vi "BLM Control Com.vi"(1 "command text in":string[](array[string]), 2 "option":T2) -> (0 "Command text out":string[][](array[string]))   [LabVIEW 2024]
uses:
  Ctl/option.ctl
  BLM Control.ctl
panel:
  in  "BLM Control":T1={"extra wait"=0, "Stepper Value"=1e-09, "Value 1"=1.0, "Value 2"=1.0, "String 1"="", "String 2"=""} {"Value 2" format="%#_6e"; "Value 1" format="%<%H:%M:%S>t"; "extra wait" min=0; "Stepper Value" step=0.045 format="%#.7e"}
  in  "cancel":bool
  in  "enter":bool
  # "BLM (Brushless Motor) Control"
  # "(BLM_ManualControl.vi needs to be open before using this program)"
  # "Distance:"
  # "deg of BLM:"
  # "seconds"
  # "AND wait extra"
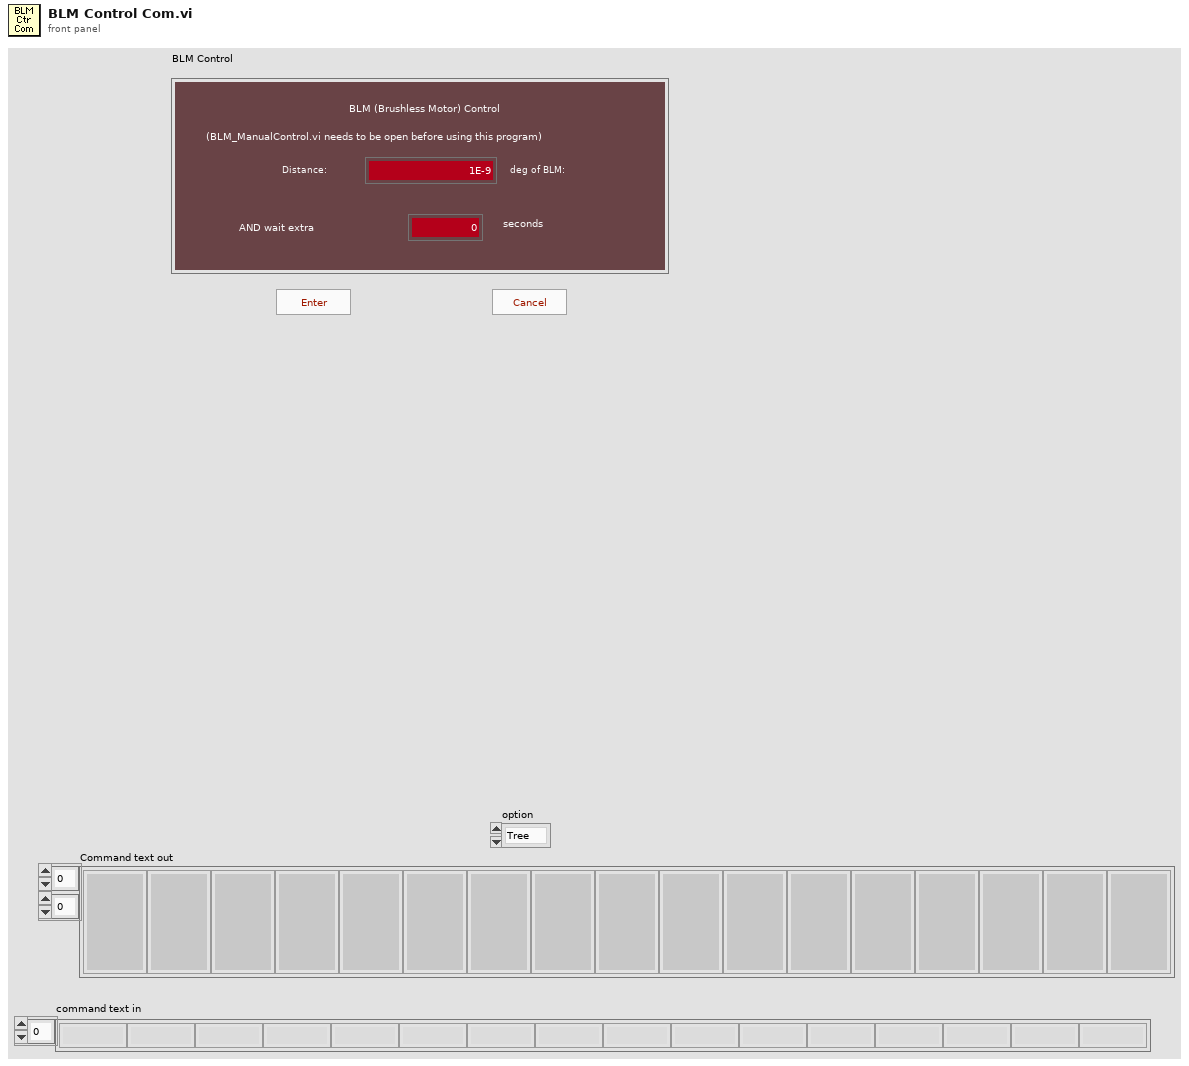
[diagram p1: front panel]
types:
  T1 = typedef "BLM Control.ctl" = cluster{"extra wait":i32, "Stepper Value":dbl, "Value 1":dbl, "Value 2":dbl, "String 1":string, "String 2":string}
  T2 = typedef "option.ctl" = enum16{"Tree", "List"}
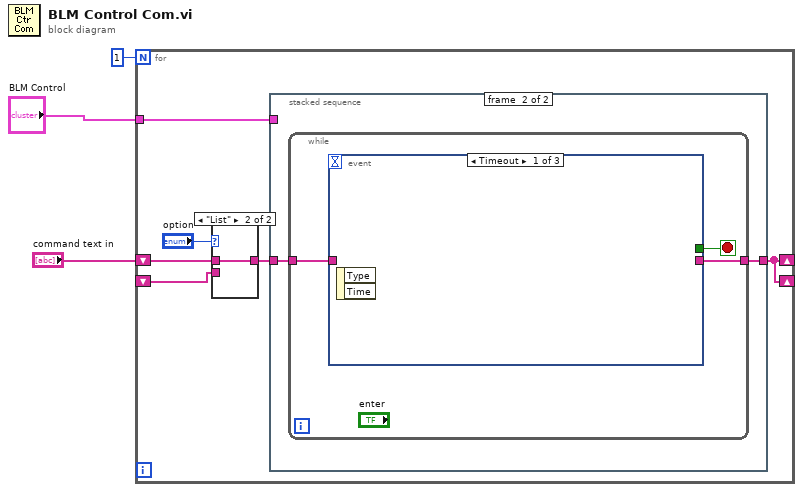
[diagram p0: block diagram]
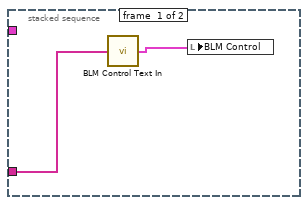
[diagram p3: hidden frame]
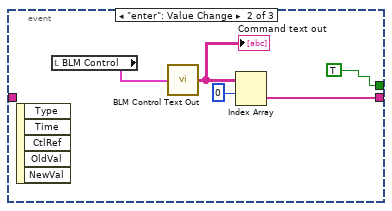
[diagram p4: hidden frame]
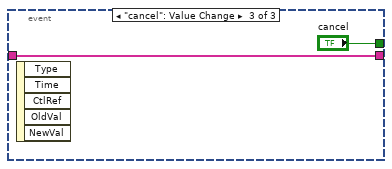
[diagram p5: hidden frame]
diagram:
  n1 = for {
    N: 1 -> [_]
    shift-right: [w4] -> _
    shift-left: _ -> [w8]
    shift-right: [w4] -> _
    shift-left: "command text in" -> [w7]
    tunnel: "BLM Control" -> [w5]
    n2 = case shown="\"List\"" "option" {
      tunnel: [w10 w11] -> w9
      tunnel: w8 -> [w10 _]
      tunnel: w7 -> [_ w11]
      frame "Tree", Default {
      }
      frame "List" {
      }
    }
    n3 = stacked-sequence {
      tunnel: [_ w15] -> w4
      tunnel: w9 -> [w12 w14]
      tunnel: w5 -> [_ _]
      frame #0 {
        n4 = call "BLM Control Text In.vi"("command text in"=w12) -> ("BLM Control"=w13:T1)
        n5 = local write "BLM Control"(w13) -> ()
      }
      frame #1 {
        n6 = while {
          tunnel: [w17] -> w15
          tunnel: w14 -> [w16]
          stop <- w18 stop-if-true
          n7 = event shown="[0] Timeout" {
            selector: _ -> [_ _ _]
            dyn-events: _ -> [_ _ _]
            timeout: _ -> [_ _ _]
            tunnel: [_ TRUE "cancel"] -> w18
            tunnel: [_ w21 w24] -> w17
            tunnel: w16 -> [_ _ w24]
            event Timeout {
              n8 = event-data() -> ()  [unwired: 1 in, 2 out]
            }
            event "enter": Value Change {
              n9 = event-data() -> ()  [unwired: 1 in, 5 out]
              n10 = local read "BLM Control"() -> (w23:T1)
              n11 = call "BLM Control Text Out.vi"("BLM Control"=w23) -> ("Command text"=w22:string[][])
              "Command text out" <- w22
              n12 = Index Array(array=w22, index (row)=0 ("disabled index (col)")) -> (element=w21:string[])  [unwired: 1 in]
            }
            event "cancel": Value Change {
              n13 = event-data() -> ()  [unwired: 1 in, 5 out]
            }
          }
        }
      }
    }
  }
